vi "Printer Comm Status.vi"(8 "error in (no error)":errorcluster, 11 "Zebra_Printer.lvclass":refnum<class "Zebra_Printer.lvclass">) -> (0 "error out":errorcluster)   [LabVIEW 2021]
uses:
  Device Manager/Printer/Sub VIs/Zebra Printer/Zebra_Printer/Zebra_Printer.lvclass
  C:/Users/enProducts/Downloads/KIA_Enproducts/KIA_Enproducts/Device Manager/DUT CAN/Controls/DUT Comm Status.ctl
  Gen fgv action.ctl
  C:/Users/enProducts/Downloads/KIA_Enproducts/KIA_Enproducts/Device Manager/DM Controls/Device List.ctl
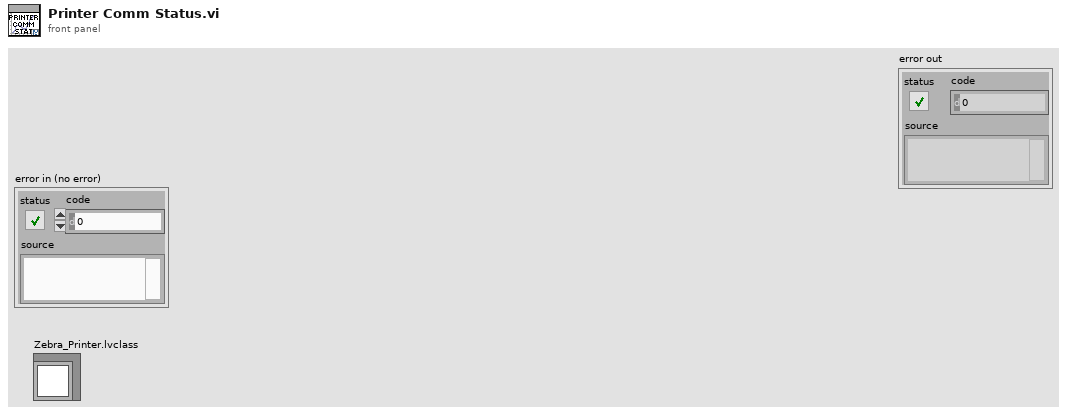
[diagram p1: front panel]
types:
  T1 = typedef "Device List.ctl" = enum16{"PLC", "Printer", "Scanner", "Screw Driver"}
  T2 = typedef "Gen FGV Action.ctl" = enum16{"Initialize", "Get Data", "Update Data", "Clear Data"}
  T3 = typedef "DUT Comm Status.ctl" = cluster{"Status":enum16{"Yet to Configure", "Configured", "Connected", "Disconnected", "Error"}, "error details":errorcluster, "Reported at":string}
  T4 = enum16{"Yet to Configure", "Configured", "Connected", "Disconnected", "Error"}
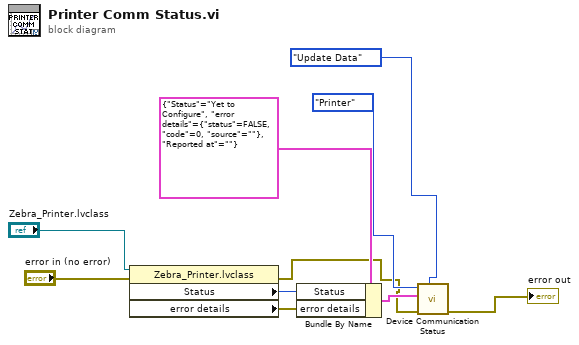
[diagram p0: block diagram]
diagram:
  n1 = property class="Zebra_Printer.lvclass"(reference="Zebra_Printer.lvclass", error in="error in (no error)") -> (error out=w3:errorcluster, "Status"=w10:T4, "error details"=w9:errorcluster)  [unwired: 1 out]
  n2 = Bundle By Name(cluster=T3 {"Status"=enum."Yet to Configure", "error details"={"status"=FALSE, "code"=0, "source"=""}, "Reported at"=""} ("DUT Communication Status"), "Status"=w10, "error details"=w9) -> (w4:T3)
  n3 = call "Device Communication Status.vi"("Action?"=Gen_FGV_Action."Update Data", "error in (no error)"=w3, "Data"=w4, "Device List"=Device_List."Printer") -> ("error out"=→"error out":errorcluster)  [unwired: 6 in, 1 out]
